vi "Interp2D zp za.vi"(4 "xy grid min":dbl[](array[numeric]), 6 "index factor (DBL)":dbl, 8 "Za array":dbl[][](array[numeric]), 9 "Zp array":dbl[][](array[numeric]), 10 "current y":dbl, 11 "current x":dbl) -> (0 "za":dbl, 3 "zp":dbl)   [LabVIEW 2010]
doc: "This VI takes in current (x,y) coordinate \"current x\" and \"current y\" and then output the distances to anterior capsule and posterior capsule based on 2D z data \"Zp array\" and \"Za array\" defined on a rectangular meshed grid (X,Y)..\nGiven current (x,y), zp and za distances are computed via 2D interpolation.\n\n\"index factor\" = (Xmax-Xmin)/size(sX) or (Ymax-Ymin)/size(Y)\n\"xy grid min\" = [Xmin Ymin]"
uses:
  Library/KevinLibraryAll/labview/KevLib01.lvlib
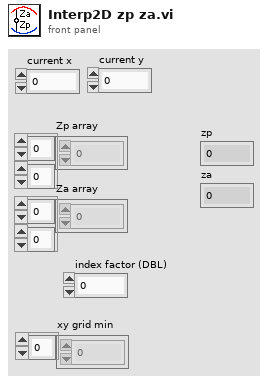
[diagram p1: front panel]
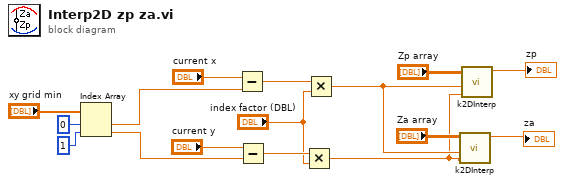
[diagram p0: block diagram]
diagram:
  n1 = Index Array(array="xy grid min", index #1=0 ("index"), index #2=1 ("index")) -> (element #1=w11:dbl, element #2=w10:dbl)
  n2 = Subtract(x="current x", y=w11) -> (x-y=w9:dbl)
  n3 = Subtract(x="current y", y=w10) -> (x-y=w8:dbl)
  n4 = Multiply(x=w8, y="index factor (DBL)") -> (x*y=w5:dbl)
  n5 = Multiply(x=w9, y="index factor (DBL)") -> (x*y=w6:dbl)
  n6 = call "k2DInterp.vi"("col"=w5, "row"=w6, "Array"="Za array") -> ("result"=→"za":dbl)  [unwired: 8 in]
  n7 = call "k2DInterp.vi"("col"=w5, "row"=w6, "Array"="Zp array") -> ("result"=→"zp":dbl)  [unwired: 8 in]
